vi "UpdateData.vi"(6 "50mA Spectra":cluster{"Wavelength":dbl[], "EL Spectrum":dbl[]}, 7 "20mA Spectra":cluster{"Wavelength":dbl[], "EL Spectrum":dbl[]}, 8 "error in (no error)":errorcluster, 10 "Data In":T1 {"50mA Data"."Current,mA" format="%_6g"; "50mA Data"."WL" format="%_6g"; "50mA Data"."Voltage" format="%_6g"; "50mA Data"."Power" format="%_6g"; "20mA Data"."Reverse" format="%#_3g"; "20mA Data"."Current,mA" format="%_6g"; "20mA Data"."Knee Current" format="%#_3g"; "20mA Data"."WL" format="%_6g"; "20mA Data"."Voltage" format="%_6g"; "20mA Data"."Power" format="%_5g"}, 11 "LotData in":refnum<class "LotData.lvclass">) -> (0 "error out":errorcluster, 2 "Db Message":string, 3 "LotData out":refnum<class "LotData.lvclass">)   [LabVIEW 2012, in "LotData.lvclass"]
uses:
  LotData.lvclass
  Controls/TestData.ctl
  Controls/LotData_Current.ctl
  LotData.lvclass/LotData.ctl
panel:
  out "Error":bool
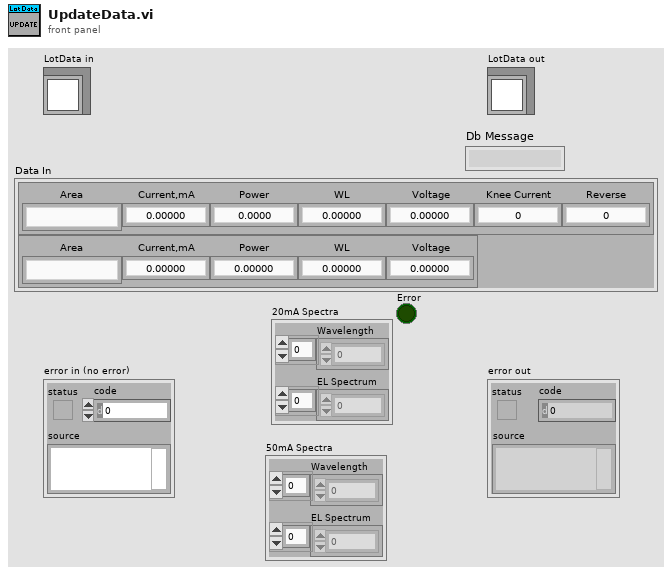
[diagram p1: front panel]
types:
  T1 = typedef "TestData.ctl" = cluster{"20mA Data":cluster{"Area":string, "Current,mA":dbl, "Power":dbl, "WL":dbl, "Voltage":dbl, "Knee Current":dbl, "Reverse":dbl}, "50mA Data":cluster{"Area":string, "Current,mA":dbl, "Power":dbl, "WL":dbl, "Voltage":dbl}}
  T2 = cluster{"Area":string, "Current,mA":dbl, "Power":dbl, "WL":dbl, "Voltage":dbl, "Knee Current":dbl, "Reverse":dbl}
  T3 = cluster{"Area":string, "Current,mA":dbl, "Power":dbl, "WL":dbl, "Voltage":dbl}
  T4 = cluster{"wl":dbl, "power":dbl, "voltage":dbl, "knee":dbl, "reverse":dbl}
  T5 = typedef "LotData.lvclass/LotData_Current.ctl" = cluster{"area":i32, "Data":cluster{"wl":dbl, "power":dbl, "voltage":dbl, "knee":dbl, "reverse":dbl}}
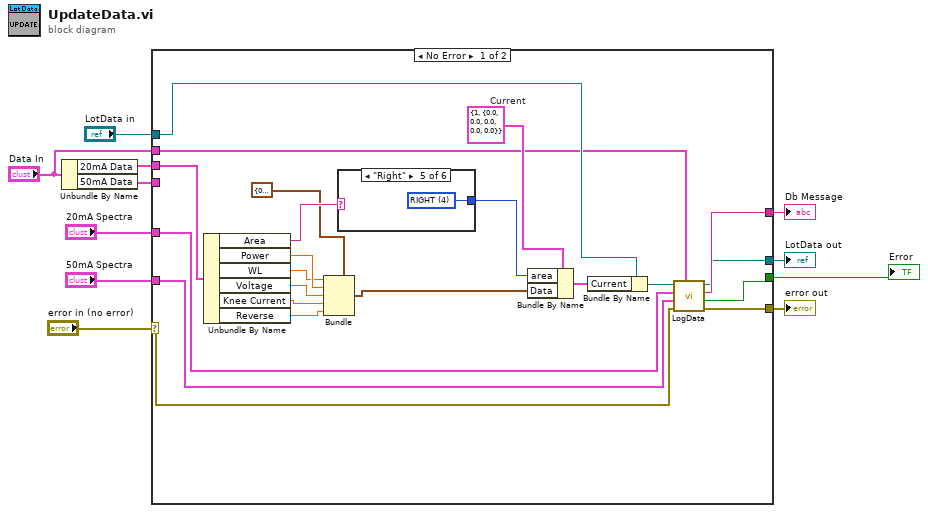
[diagram p0: block diagram]
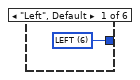
[diagram p2: hidden frame]
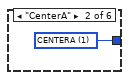
[diagram p3: hidden frame]
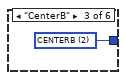
[diagram p4: hidden frame]
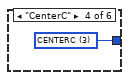
[diagram p5: hidden frame]
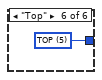
[diagram p6: hidden frame]
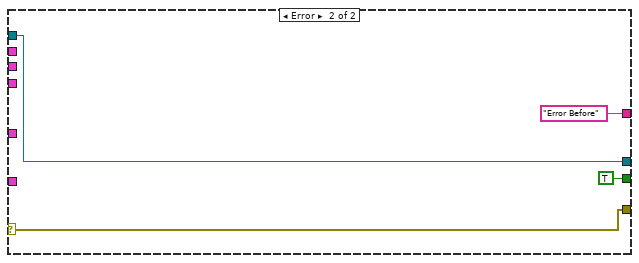
[diagram p7: hidden frame]
diagram:
  n1 = Unbundle By Name("Data In") -> ("20mA Data"=w9:T2, "50mA Data"=w8:T3)
  n2 = case shown="No Error" "error in (no error)" {
    selector: "error in (no error)" -> [w25 w43]
    tunnel: [w14 w43] -> w6
    tunnel: [w15 w42] -> w7
    tunnel: "LotData in" -> [w22 w42]
    tunnel: w9 -> [w31 _]
    tunnel: w8 -> [_ _]
    tunnel: "20mA Spectra" -> [w16 _]
    tunnel: "50mA Spectra" -> [w21 _]
    tunnel: [w24 "Error Before" ("LogData")] -> w3
    tunnel: [w13 TRUE ("Error")] -> w2
    tunnel: "Data In" -> [w12 _]
    frame No Error {
      w33 = T5 {"area"=1, "Data"={"wl"=0.0, "power"=0.0, "voltage"=0.0, "knee"=0.0, "reverse"=0.0}}  # Current
      n3 = Unbundle By Name(w31) -> ("Area"=w30:string, "Power"=w29:dbl, "WL"=w28:dbl, "Voltage"=w27:dbl, "Knee Current"=w26:dbl, "Reverse"=w19:dbl)
      n4 = Bundle(cluster=T4 {"wl"=0.0, "power"=0.0, "voltage"=0.0, "knee"=0.0, "reverse"=0.0} ("Data"), "wl"=w28, "power"=w29, "voltage"=w27, "knee"=w26, "reverse"=w19) -> (w17:T4)
      n5 = case shown="\"Right\"" w30 {
        tunnel: [w34 w35 w36 w37 w38 w39] -> w20
        frame "Left", Default {
          w34 = 6 items=["CENTERA"=1, "CENTERB"=2, "CENTERC"=3, "RIGHT"=4, "TOP"=5, "LEFT"=6] ("area")
        }
        frame "CenterA" {
          w35 = 1 items=["CENTERA"=1, "CENTERB"=2, "CENTERC"=3, "RIGHT"=4, "TOP"=5, "LEFT"=6] ("area")
        }
        frame "CenterB" {
          w36 = 2 items=["CENTERA"=1, "CENTERB"=2, "CENTERC"=3, "RIGHT"=4, "TOP"=5, "LEFT"=6] ("area")
        }
        frame "CenterC" {
          w37 = 3 items=["CENTERA"=1, "CENTERB"=2, "CENTERC"=3, "RIGHT"=4, "TOP"=5, "LEFT"=6] ("area")
        }
        frame "Right" {
          w38 = 4 items=["CENTERA"=1, "CENTERB"=2, "CENTERC"=3, "RIGHT"=4, "TOP"=5, "LEFT"=6] ("area")
        }
        frame "Top" {
          w39 = 5 items=["CENTERA"=1, "CENTERB"=2, "CENTERC"=3, "RIGHT"=4, "TOP"=5, "LEFT"=6] ("area")
        }
      }
      n6 = Bundle By Name(cluster=w33, "area"=w20, "Data"=w17) -> (w32:T5)
      n7 = Bundle By Name(cluster=w22, "Current"=w32) -> (w23:refnum<class "LotData.lvclass">)
      n8 = call-dynamic "LogData.vi"("LotData in"=w23, "20mA Spectra"=w16, "50mA Spectra"=w21, "error in (no error)"=w25, "Data In"=w12) -> ("LotData out"=w15:refnum<class "LotData.lvclass">, "LogData"=w24:string, "Error"=w13:bool, "error out"=w14:errorcluster)  [unwired: 2 in]
    }
    frame Error {
    }
  }
  "error out" <- w6
  "LotData out" <- w7
  "Db Message" <- w3
  "Error" <- w2
